vi "FeatureHasher.vi"(8 "error in":errorcluster caption="entrée d'erreur", 11 "FeatureHasher":T1={"n_features"=1048576, "input_type"="dict", "dtype"="float", "alternate_sign"=TRUE}) -> (0 "error out":errorcluster caption="sortie d'erreur", 3 "FeatureHasher.lvclass":refnum<class "FeatureHasher.lvclass">)   [LabVIEW 2020]
doc: "Implements feature hashing, aka the hashing trick.\n\nThis class turns sequences of symbolic feature names (strings) into scipy.sparse matrices, using a hash function to compute the matrix column corresponding to a name. The hash function employed is the signed 32-bit version of Murmurhash3.\n\nFeature names of type byte string are used as-is. Unicode strings are converted to UTF-8 first, but no Unicode normalization is done. Feature values must be (finite) numbers.\n\nThis class is a low-memory alternative to DictVectorizer and CountVectorizer, intended for large-scale (online) learning and situations where memory is tight, e.g. when running prediction code on embedded devices.\n\nParameters : \n\n- n_features : int, default=2**20\nThe number of features (columns) in the output matrices. Small numbers of features are likely to cause hash collisions, but large numbers will cause larger coefficient dimensions in linear learners.\n\n- input_type : {“dict”, “pair”}, default=”dict”\nEither “dict” (the default) to accept dictionaries over (feature_name, value); “pair” to accept pairs of (feature_name, value); or “string” to accept single strings. feature_name should be a string, while value should be a number. In the case of “string”, a value of 1 is implied. The feature_name is hashed to find the appropriate column for the feature. The value’s sign might be flipped in the output (but see non_negative, below).\n\n- dtype : numpy dtype, default=np.float64\nThe type of feature values. Passed to scipy.sparse matrix constructors as the dtype argument. Do not set this to bool, np.boolean or any unsigned integer type.\n\n- alternate_sign : bool, default=True\nWhen True, an alternating sign is added to the features as to approximately conserve the inner product in the hashed space even for small n_features. This approach is similar to sparse random projection.\n\n\n\nMethods : \n\n\n- Fit : No-op. This method doesn’t do anything. It exists purely for compatibility with the scikit-learn transformer API.\n\nParameters : X : ndarray\n\nReturns : String : OK\n\n\n- Fit Transform : Fit to data, then transform it. Fits transformer to X and y with optional parameters fit_params and returns a transformed version of X.\n\nParameters : X : {array-like, sparse matrix, dataframe} of shape (n_samples, n_features)\n y : ndarray of shape (n_samples,), default=None\n Target values\n\nReturns : X_new : ndarray array of shape (n_samples, n_features_new)\n Transformed array.\n\n\n-Transform : Transform a sequence of instances to a scipy.sparse matrix.\n\nParameters : X : iterable over iterable over raw features, length = n_samples\n Samples. Each sample must be iterable an (e.g., a list or tuple) containing/generating feature names (and optionally values, see the input_type constructor argument) which will be hashed. raw_X need not support the len function, so it can be the result of a generator; n_samples is determined on the fly.\n\nReturns : X : sparse matrix of shape (n_samples, n_features)\n Feature matrix, for use with estimators or further transformers."
uses:
  FeatureHasher.lvclass
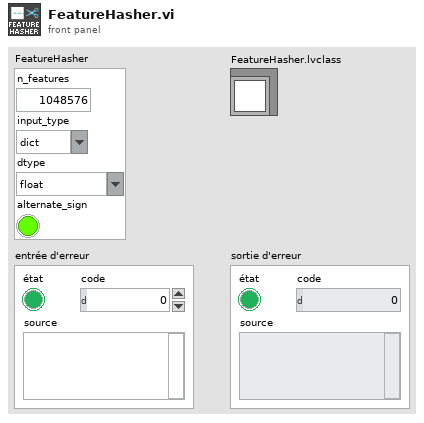
[diagram p1: front panel]
types:
  T1 = cluster{"n_features":i32, "input_type":string, "dtype":string, "alternate_sign":bool}
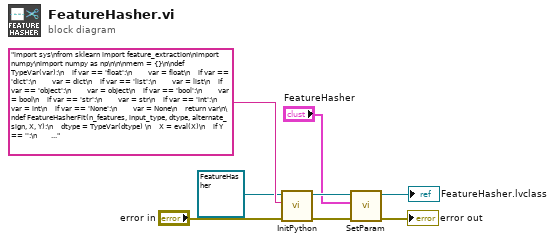
[diagram p0: block diagram]
diagram:
  n1 = call-dynamic "InitPython.vi"("error in (no error)"="error in", "Python Instruction"="import sys\nfrom sklearn import feature_extraction\nimport numpy\nimport numpy as np\n\n\nmem = {}\n\ndef TypeVar(var):\n    if var == 'float':\n        var = float\n    if var == 'dict':\n        var = dict\n    if var == 'list':\n        var = list\n    if var == 'object':\n        var = object\n    if var == 'bool':\n        var = bool\n    if var == 'str':\n        var = str\n    if var == 'int':\n        var = int\n    if var == 'None':\n        var = None\n    return var\n\ndef FeatureHasherFit(n_features, input_type, dtype, alternate_sign, X, Y):\n    dtype = TypeVar(dtype) \n    X = eval(X)\n    if Y == '':\n        Y = None\n    else:\n        Y = eval(Y)\n    try:\n        FeatureHasher = feature_extraction.FeatureHasher(n_features, input_type, dtype, alternate_sign).fit(X, Y)\n        mem['FitFeatureHasher'] = FeatureHasher\n        return str('OK')\n    except:\n        erreur = sys.exc_info()\n        typerr = u\"%s\" % (erreur[0])\n        typerr = typerr[typerr.find(\"'\")+1:typerr.rfind(\"'\")]\n        msgerr = u\"%s\" % (erreur[1])\n        message = str('/!\\\\ {0} : {1}'. format(typerr,msgerr))\n        return message \n\ndef FeatureHasherFitTransform(n_features, input_type, dtype, alternate_sign, X, Y):\n    dtype = TypeVar(dtype)   \n    X = eval(X)\n    if Y == '':\n        Y = None\n    else:\n        Y = eval(Y)\n    try:\n        FeatureHasher = feature_extraction.FeatureHasher(n_features, input_type, dtype, alternate_sign).fit_transform(X, Y)\n        dtype = type(FeatureHasher)\n        if dtype == numpy.ndarray:\n            FeatureHasher = FeatureHasher.tolist()\n            return str(FeatureHasher)\n        else:\n            Mat = FeatureHasher.tocoo()\n            return str(list(zip(Mat.row, Mat.col, Mat.data)))\n    except:\n        erreur = sys.exc_info()\n        typerr = u\"%s\" % (erreur[0])\n        typerr = typerr[typerr.find(\"'\")+1:typerr.rfind(\"'\")]\n        msgerr = u\"%s\" % (erreur[1])\n        message = str('/!\\\\ {0} : {1}'. format(typerr,msgerr))\n        return message \n    \ndef FeatureHasherTransform(n_features, input_type, dtype, alternate_sign, X, Y):\n    dtype = TypeVar(dtype)    \n    X = eval(X)\n    if Y == '':\n        Y = None\n    else:\n        Y = eval(Y)\n    try:\n        FeatureHasher = mem['FitFeatureHasher'].transform(X, Y)\n        dtype = type(FeatureHasher)\n        if dtype == numpy.ndarray:\n            FeatureHasher = FeatureHasher.tolist()\n            return str(FeatureHasher)\n        else:\n            Mat = FeatureHasher.tocoo()\n            return str(list(zip(Mat.row, Mat.col, Mat.data)))\n    except:\n        erreur = sys.exc_info()\n        typerr = u\"%s\" % (erreur[0])\n        typerr = typerr[typerr.find(\"'\")+1:typerr.rfind(\"'\")]\n        msgerr = u\"%s\" % (erreur[1])\n        message = str('/!\\\\ {0} : {1}'. format(typerr,msgerr))\n        return message", "Scikit-learn en entrée"=refnum<class "FeatureHasher.lvclass"> refnum ("FeatureHasher.lvclass")) -> ("error out"=w1:errorcluster, "Scikit-learn en sortie"=w5:refnum<class "FeatureHasher.lvclass">)  [unwired: 7 in]
  n2 = call-dynamic "SetParam.vi"("error in (no error)"=w1, "FeatureHasher"="FeatureHasher", "FeatureHasher.lvclass"=w5) -> ("error out"=→"error out":errorcluster, "FeatureHasher.lvclass"=→"FeatureHasher.lvclass":refnum<class "FeatureHasher.lvclass">)  [unwired: 7 in]
